vi "RLC_fake.vi"(3 "f2 [Hz]":dbl format="%#_6p", 4 "f1 [Hz]":dbl format="%#_6p", 5 "Rp [Ohm]":dbl format="%#_6p", 6 "f [Hz]":dbl format="%#_6p") -> (0 "Z":dbl format="%#_6p", 1 "Xs":dbl format="%#_6p", 2 "Rs":dbl format="%#_6p")   [LabVIEW 2013]
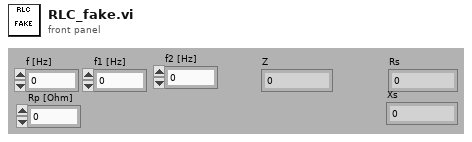
[diagram p1: front panel]
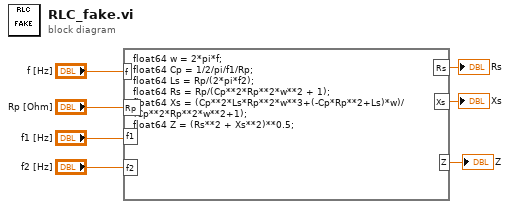
[diagram p0: block diagram]
diagram:
  n1 = formula code="float64 w = 2*pi*f;\nfloat64 Cp = 1/2/pi/f1/Rp;\nfloat64 Ls = Rp/(2*pi*f2);\nfloat64 Rs = Rp/(Cp**2*Rp**2*w**2 + 1);\nfloat64 Xs = (Cp**2*Ls*Rp**2*w**3+(-Cp*Rp**2+Ls)*w)/(Cp**2*Rp**2*w**2+1);\nfloat64 Z = (Rs**2 + Xs**2)**0.5;"("f"="f [Hz]", "Rp"="Rp [Ohm]", "f1"="f1 [Hz]", "f2"="f2 [Hz]") -> ("Rs"=→"Rs":dbl, "Xs"=→"Xs":dbl, "Z"=→"Z":dbl)
